vi "RSZVB Get Trace Display State.vi"(8 "error in (no error)":errorcluster {"code" format="%.0x"}, 9 "Single Trace Name (\"Trc1\")":string="Trc1", 10 "Trace Type (0)":i32(ring) items=["All Data Traces", "All Memory Traces", "Single Trace"], 11 "VISA session":refnum<visa-resource-name>) -> (0 "error out":errorcluster {"code" format="%.0x"}, 1 "Show Trace":bool, 3 "dup VISA session":refnum<visa-resource-name>)   [LabVIEW 2011]
doc: "This VI returns whether the trace is shown or not.\n\nRemote-control command(s):\nDISPlay[:WINDow<Wnd>]:TRACe<WndTr>:SHOW? DALL | MALL | '<trace_name>'"
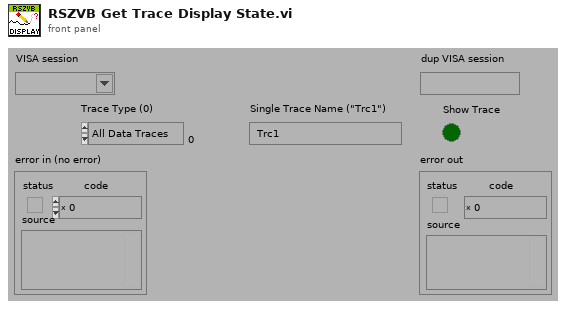
[diagram p1: front panel]
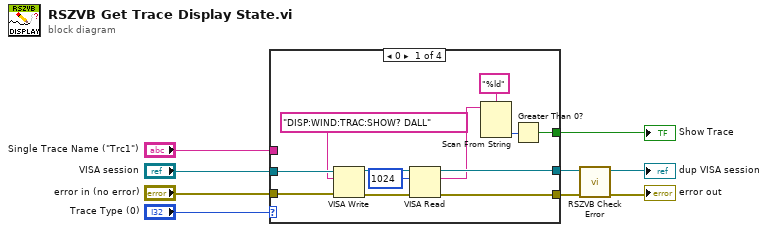
[diagram p0: block diagram]
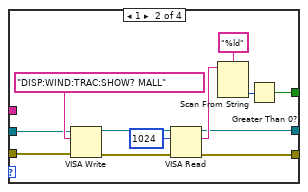
[diagram p2: hidden frame]
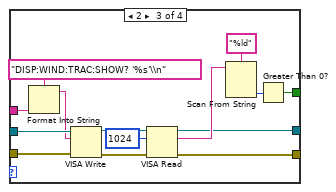
[diagram p3: hidden frame]
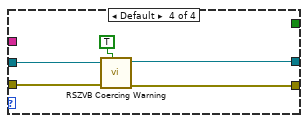
[diagram p4: hidden frame]
diagram:
  n1 = case shown="0" "Trace Type (0)" {
    tunnel: "VISA session" -> [w21 w26 w41 w51]
    tunnel: "error in (no error)" -> [w20 w25 w40 w52]
    tunnel: [w15 w24 w39 w49] -> w5
    tunnel: [w14 w23 w38 w48] -> w3
    tunnel: [w10 w22 w37 _] -> w6
    tunnel: "Single Trace Name (\"Trc1\")" -> [_ _ w35 _]
    frame 0 {
      n2 = VISA Write(VISA resource name=w21, write buffer="DISP:WIND:TRAC:SHOW? DALL", error in (no error)=w20) -> (VISA resource name out=w17:refnum<visa-resource-name>, error out=w18:errorcluster)  [unwired: 1 out]
      n3 = VISA Read(VISA resource name=w17, byte count=u32 1024, error in (no error)=w18) -> (VISA resource name out=w14:refnum<visa-resource-name>, read buffer=w12:string, error out=w15:errorcluster)  [unwired: 1 out]
      n4 = Scan From String(format string="%ld", input string=w12) -> (output 1=w11:i32)  [unwired: 3 in, 3 out]
      n5 = Greater Than 0?(x=w11) -> (x > 0?=w10:bool)
    }
    frame 1 {
      n6 = VISA Write(VISA resource name=w26, write buffer="DISP:WIND:TRAC:SHOW? MALL", error in (no error)=w25) -> (VISA resource name out=w31:refnum<visa-resource-name>, error out=w32:errorcluster)  [unwired: 1 out]
      n7 = VISA Read(VISA resource name=w31, byte count=u32 1024, error in (no error)=w32) -> (VISA resource name out=w23:refnum<visa-resource-name>, read buffer=w28:string, error out=w24:errorcluster)  [unwired: 1 out]
      n8 = Scan From String(format string="%ld", input string=w28) -> (output 1=w27:i32)  [unwired: 3 in, 3 out]
      n9 = Greater Than 0?(x=w27) -> (x > 0?=w22:bool)
    }
    frame 2 {
      n10 = Format Into String(format string="DISP:WIND:TRAC:SHOW? '%s'\\n", w35) -> (resulting string=w34:string)  [unwired: 2 in, 1 out]
      n11 = VISA Write(VISA resource name=w41, write buffer=w34, error in (no error)=w40) -> (VISA resource name out=w46:refnum<visa-resource-name>, error out=w47:errorcluster)  [unwired: 1 out]
      n12 = VISA Read(VISA resource name=w46, byte count=u32 1024, error in (no error)=w47) -> (VISA resource name out=w38:refnum<visa-resource-name>, read buffer=w43:string, error out=w39:errorcluster)  [unwired: 1 out]
      n13 = Scan From String(format string="%ld", input string=w43) -> (output 1=w42:i32)  [unwired: 3 in, 3 out]
      n14 = Greater Than 0?(x=w42) -> (x > 0?=w37:bool)
    }
    frame Default {
      n15 = call "RSZVB Coercing Warning.vi"("In Range?"=TRUE, "error in (no error)"=w52, "VISA session"=w51) -> ("error out"=w49:errorcluster, "dup VISA session"=w48:refnum<visa-resource-name>)  [unwired: 7 in]
    }
  }
  "Show Trace" <- w6
  n16 = call "RSZVB Check Error.vi"("error in (no error)"=w5, "VISA session"=w3) -> ("error out"=→"error out":errorcluster, "dup VISA session"=→"dup VISA session":refnum<visa-resource-name>)  [unwired: 8 in]
